vi "addConditionalDisableAroundCLFN.vi"() -> ()   [LabVIEW 2016]
panel:
  in  "Path":path=path "C:/LSST_TS/SystemSW/ts_sallabviewrt_tools/ts_sallv_exa/VIs/EXA_Connect.vi"
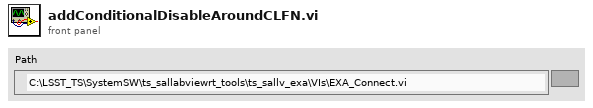
[diagram p1: front panel]
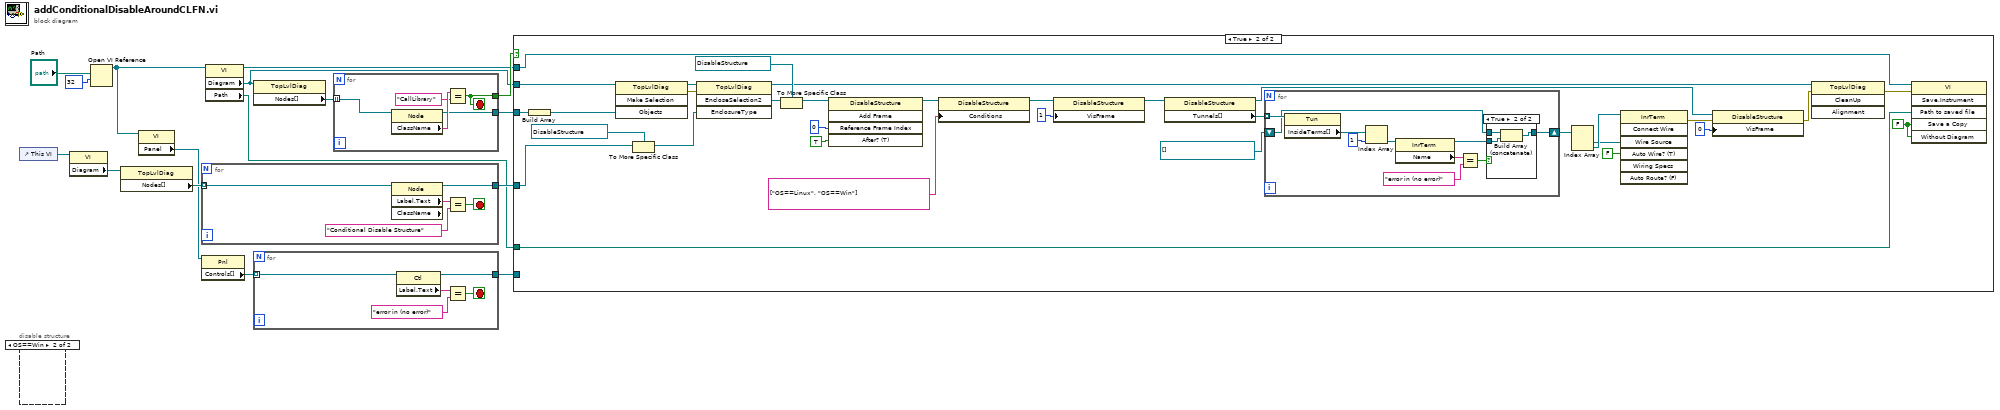
[diagram p0: block diagram]
diagram:
  n1 = control-ref of="This VI"() -> (w8:refnum<vi>)
  n2 = disable-structure "Conditional Disable Structure" shown="OS==Win" {
    frame condition #0 {
    }
    frame condition #1 (active) {
    }
  }
  n3 = property on="Property Node" class="VI"(reference=w8) -> ("Diagram"=w9:refnum<vi>)  [unwired: 1 in, 2 out]
  n4 = Open VI Reference(vi path="Path", options=32) -> (vi reference=w5:refnum<vi>)  [unwired: 4 in, 1 out]
  n5 = property on="Property Node" class="TopLvlDiag"(reference=w9) -> ("Nodes[]"=w10:refnum<vi>[])  [unwired: 1 in, 2 out]
  n6 = property on="Property Node" class="VI"(reference=w5) -> ("Panel"=w7:refnum<vi>)  [unwired: 1 in, 2 out]
  n7 = for {
    tunnel: w10 -> [w21] mode=indexing
    tunnel: [w18] -> w11
    stop <- w19 stop-if-true
    n8 = property class="Node" props=["Label", "Text", "ClassName"](reference=w21) -> (reference out=w18:refnum<vi>, "Label.Text"=w17:string)  [unwired: 1 in, 2 out]
    n9 = Equal?(x=w17, y="Conditional Disable Structure" ("Class Name")) -> (x = y?=w19:bool)
  }
  n10 = property on="Property Node" class="Pnl"(reference=w7) -> ("Controls[]"=w6:refnum<vi>[])  [unwired: 1 in, 2 out]
  n11 = property on="Property Node" class="VI"(reference=w5) -> (reference out=w3:refnum<vi>, "Diagram"=w12:refnum<vi>, "Path"=w2:path)  [unwired: 1 in, 1 out]
  n12 = property on="Property Node" class="TopLvlDiag"(reference=w12) -> ("Nodes[]"=w15:refnum<vi>[])  [unwired: 1 in, 2 out]
  n13 = for {
    tunnel: w6 -> [w26] mode=indexing
    tunnel: [w24] -> w4
    stop <- w22 stop-if-true
    n14 = property class="Ctl"(reference=w26) -> (reference out=w24:refnum<vi>, "Label.Text"=w23:string)  [unwired: 1 in, 1 out]
    n15 = Equal?(x=w23, y="error in (no error)" ("Class Name")) -> (x = y?=w22:bool)
  }
  n16 = for {
    tunnel: w15 -> [w31] mode=indexing
    tunnel: [w28] -> w14
    tunnel: [w27] -> w13
    stop <- w28 stop-if-true
    n17 = property class="Node"(reference=w31) -> (reference out=w27:refnum<vi>, "ClassName"=w30:string)  [unwired: 1 in, 1 out]
    n18 = Equal?(x=w30, y="CallLibrary" ("Class Name")) -> (x = y?=w28:bool)
  }
  n19 = case shown="True" w14 {
    tunnel: w13 -> [_ w63]
    tunnel: w12 -> [_ w64]
    tunnel: w11 -> [_ w59]
    tunnel: w4 -> [_ _]
    tunnel: w3 -> [_ w35]
    tunnel: w2 -> [_ w32]
    frame False {
    }
    frame True {
      w33 = FALSE ("Save a Copy")
      n20 = Build Array(w63) -> (w62:refnum<vi>[])
      n21 = invoke class="TopLvlDiag" method="Make Selection"(reference=w64, "Objects"=w62) -> (reference out=w61:refnum<vi>, error out=w60:errorcluster)  [unwired: 2 in, 2 out]
      n22 = To More Specific Class(target class=refnum<vi> refnum ("EnclosureType"), reference=w59) -> (specific class reference=w57:refnum<vi>)  [unwired: 1 in, 1 out]
      n23 = invoke class="TopLvlDiag" method="EncloseSelection2"(reference=w61, error in=w60, "EnclosureType"=w57) -> (reference out=w37:refnum<vi>, "EncloseSelection2"=w55:refnum<vi>)  [unwired: 1 in, 2 out]
      n24 = To More Specific Class(target class=refnum<vi> refnum ("EnclosureType"), reference=w55) -> (specific class reference=w54:refnum<vi>)  [unwired: 1 in, 1 out]
      n25 = invoke class="DisableStructure" method="Add Frame"(reference=w54, "Reference Frame Index"=u32 0, "After? (T)"=TRUE) -> (reference out=w53:refnum<vi>)  [unwired: 2 in, 4 out]
      n26 = property class="DisableStructure"(reference=w53, "Conditions"=string[] ["OS==Linux", "OS==Win"]) -> (reference out=w49:refnum<vi>)  [unwired: 1 in, 1 out]
      n27 = property class="DisableStructure"(reference=w49, "VisFrame"=i16 1 ("Active Frame")) -> (reference out=w47:refnum<vi>)  [unwired: 1 in, 1 out]
      n28 = property class="DisableStructure"(reference=w47) -> (reference out=w40:refnum<vi>, "Tunnels[]"=w46:refnum<vi>[])  [unwired: 1 in, 1 out]
      n29 = for {
        tunnel: w46 -> [w74] mode=indexing
        shift-right: [w66] -> w44
        shift-left: refnum<vi>[] [] ("Array 6") -> [w68]
        n30 = property class="Tun"(reference=w74) -> ("InsideTerms[]"=w73:refnum<vi>[])  [unwired: 1 in, 2 out]
        n31 = Index Array(array=w73, index=1) -> (element=w71:refnum<vi>)
        n32 = property class="InrTerm"(reference=w71) -> (reference out=w65:refnum<vi>, "Name"=w70:string)  [unwired: 1 in, 1 out]
        n33 = Equal?(x=w70, y="error in (no error)") -> (x = y?=w67:bool)
        n34 = case shown="True" w67 {
          tunnel: w68 -> [w75 w78]
          tunnel: [w75 w77] -> w66
          tunnel: w65 -> [_ w76]
          frame False {
          }
          frame True {
            n35 = Build Array (concatenate)(w78, w76) -> (w77:refnum<vi>[])
          }
        }
      }
      n36 = Index Array(array=w44) -> (element #1=w42:refnum<vi>, element #2=w43:refnum<vi>)  [unwired: 2 in]
      n37 = invoke class="InrTerm" method="Connect Wire"(reference=w43, "Wire Source"=w42, "Auto Wire? (T)"=FALSE) -> (error out=w38:errorcluster)  [unwired: 4 in, 6 out]
      n38 = property class="DisableStructure"(reference=w40, error in=w38, "VisFrame"=u32 0 ("Visible Frame")) -> (error out=w36:errorcluster)  [unwired: 1 out]
      n39 = invoke class="TopLvlDiag" method="CleanUp"(reference=w37, error in=w36) -> (error out=w34:errorcluster)  [unwired: 2 in, 3 out]
      n40 = invoke class="VI" method="Save.Instrument"(reference=w35, error in=w34, "Path to saved file"=w32, "Save a Copy"=w33, "Without Diagram"=w33) -> ()  [unwired: 1 in, 6 out]
    }
  }
